vi "Stop All.vi"(8 "error in (no error)":errorcluster, 11 "LINX-PCA9865 PWM in":refnum<class "LINX-PCA9685 PWM.lvclass">) -> (0 "error out":errorcluster, 3 "LINX-PCA9865 PWM out":refnum<class "LINX-PCA9685 PWM.lvclass">)   [LabVIEW 2020, in "LINX-PCA9685 PWM.lvclass"]
doc: "Sends the all-stop command to turn off all PWM channels."
uses:
  LINX-PCA9685 PWM.lvclass
  LINX I2C/LINX I2C.lvclass
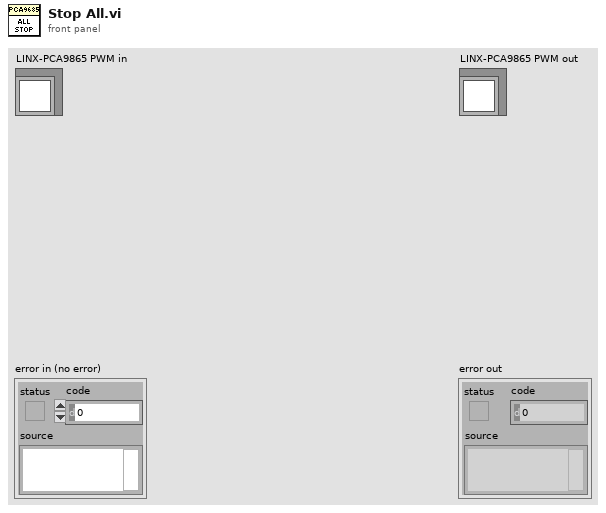
[diagram p1: front panel]
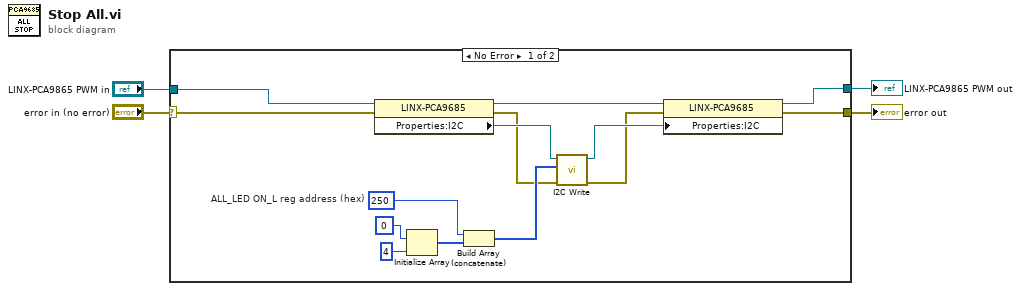
[diagram p0: block diagram]
diagram:
  n1 = case shown="No Error" "error in (no error)" {
    selector: "error in (no error)" -> [w7 w20]
    tunnel: [w5 w20] -> w3
    tunnel: [w6 w19] -> w1
    tunnel: "LINX-PCA9865 PWM in" -> [w8 w19]
    frame No Error {
      w17 = u8 250  # ALL_LED ON_L reg address (hex)
      n2 = property class="LINX-PCA9685"(reference=w8, error in=w7) -> (reference out=w13:refnum<class "LINX-PCA9685 PWM.lvclass">, error out=w9:errorcluster, "Properties:I2C"=w12:refnum<class "LINX I2C.lvclass">)
      n3 = Initialize Array(u8 0 ("I2C Slave Address 2"), 4 ("dimension size")) -> (w14:u8[])
      n4 = Build Array (concatenate)(w17, w14) -> (w18:u8[])
      n5 = call "I2C Write.vi"("error in (no error)"=w9, "Bytes to Write"=w18, "LINX I2C in"=w12) -> ("error out"=w10:errorcluster, "LINX I2C out"=w11:refnum<class "LINX I2C.lvclass">)  [unwired: 7 in]
      n6 = property class="LINX-PCA9685"(reference=w13, error in=w10, "Properties:I2C"=w11) -> (reference out=w6:refnum<class "LINX-PCA9685 PWM.lvclass">, error out=w5:errorcluster)
    }
    frame Error {
    }
  }
  "error out" <- w3
  "LINX-PCA9865 PWM out" <- w1
